vi "origin_distance (SubVI).vi"(8 "error in (no error)":errorcluster, 9 "Image Dst":T1, 10 "Origin Pixel":cluster{"X":sgl, "Y":sgl}, 11 "Image Src":T1) -> (0 "error out":errorcluster, 1 "Number of Particles":i32, 2 "Array":string[](array[string]), 3 "Array of Real World Coordinates":cluster{"X":sgl, "Y":sgl}[](array[cluster]), 5 "Image Out":T1)   [LabVIEW 2020]
uses:
  <vilib>/vision/Image Controls.llb/IMAQ Image.ctl
  <vilib>/vision/NI_Vision_Development_Module.lvlib
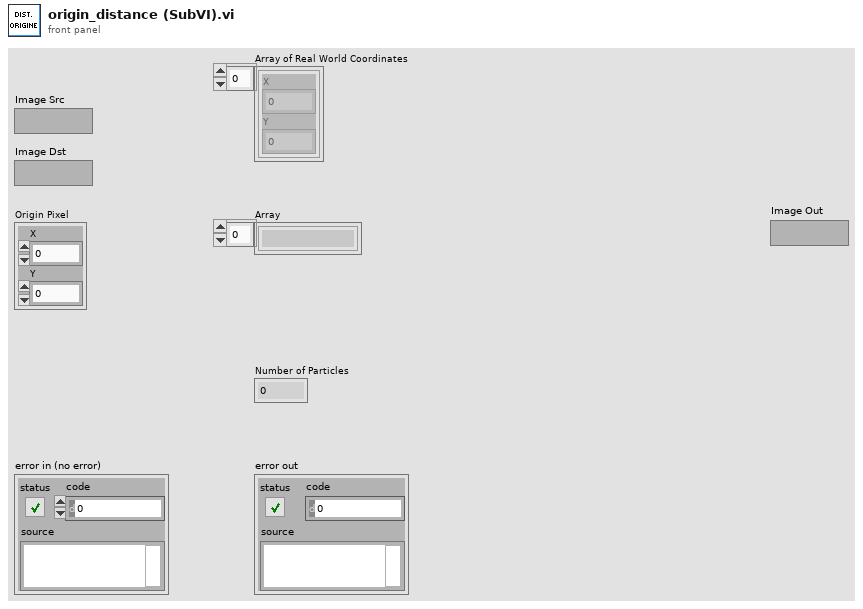
[diagram p1: front panel]
types:
  T1 = typedef "IMAQ Image.ctl" = refnum<image>
  T2 = cluster{"Area":dbl, "Number of Holes":dbl, "Bounding Rect":cluster{"Left":dbl, "Top":dbl, "Right":dbl, "Bottom":dbl}, "Center of Mass":cluster{"X":dbl, "Y":dbl}, "Orientation":dbl, "Dimensions":cluster{"Width":dbl, "Height":dbl}}[]
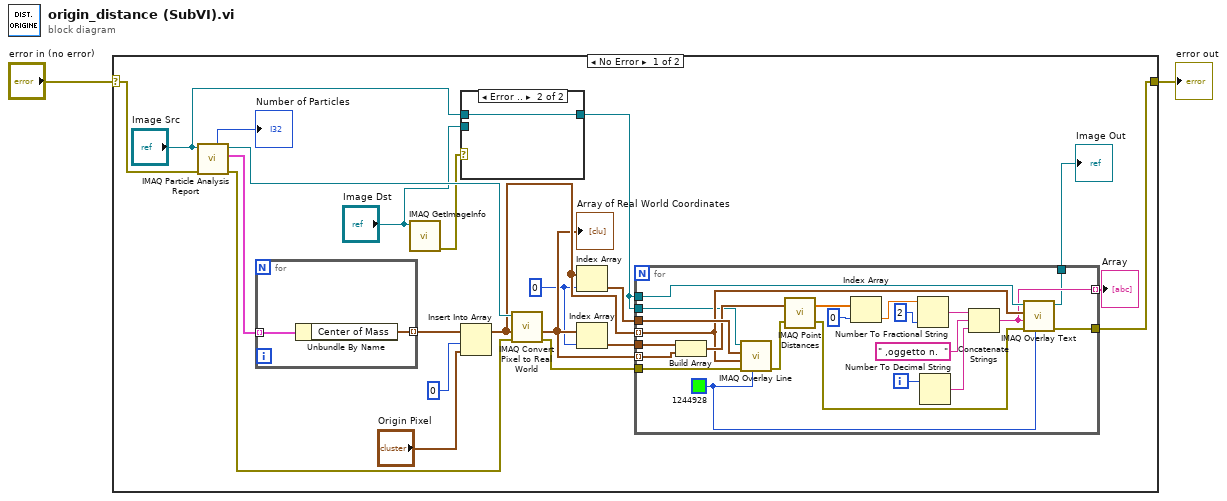
[diagram p0: block diagram]
diagram:
  n1 = case shown="No Error" "error in (no error)" {
    selector: "error in (no error)" -> [w9 w50]
    tunnel: [w8 w50] -> w1
    frame No Error {
      w12 = 0 ("index")
      n2 = call "IMAQ Particle Analysis Report"("error in (no error)"=w9, "Image"="Image Src") -> ("error out"=w21:errorcluster, "Particle Reports (Pixels)"=w19:T2, "Image Out (duplicate)"=w20:T1, "Number of Particles"=→"Number of Particles":i32)  [unwired: 4 in, 2 out]
      n3 = for {
        tunnel: [w48] -> w15 mode=indexing
        tunnel: w19 -> [w49] mode=indexing
        n4 = Unbundle By Name(w49) -> ("Center of Mass"=w48:cluster{"X":dbl, "Y":dbl})
      }
      n5 = call "IMAQ GetImageInfo"("Image"="Image Dst") -> ("error out"=w7:errorcluster)  [unwired: 3 in, 7 out]
      n6 = case shown="Error .." w7 {
        tunnel: "Image Dst" -> [w24 _]
        tunnel: [w24 w25] -> w5
        tunnel: "Image Src" -> [_ w25]
        frame No Error {
        }
        frame Error {
        }
      }
      n7 = Insert Into Array(array=w15, index=0, new element="Origin Pixel") -> (w16:cluster{"X":dbl, "Y":dbl}[])
      n8 = call "IMAQ Convert Pixel to Real World"("error in (no error)"=w21, "Array of Pixel Coordinates"=w16, "Calibrated Image"=w20) -> ("error out"=w22:errorcluster, "Array of Real World Coordinates"=w14:cluster{"X":sgl, "Y":sgl}[])  [unwired: 3 in, 4 out]
      "Array of Real World Coordinates" <- w14
      n9 = Index Array(array=w16, index=w12) -> (element=w11:cluster{"X":dbl, "Y":dbl})
      n10 = Index Array(array=w14, index=w12) -> (element=w13:cluster{"X":sgl, "Y":sgl})
      n11 = for {
        tunnel: w16 -> [w41] mode=indexing
        tunnel: w11 -> [w47]
        tunnel: w13 -> [w44]
        tunnel: w14 -> [w42] mode=indexing
        tunnel: [w45] -> w8
        tunnel: w5 -> [w30]
        tunnel: w5 -> [w29]
        tunnel: w22 -> [w28]
        tunnel: [w27] -> w23 mode=indexing
        tunnel: [w26] -> w3
        i -> [w36]
        w40 = u32 1244928 ("Color")
        n12 = Build Array(w44, w42) -> (w43:cluster{"X":sgl, "Y":sgl}[])
        n13 = call "IMAQ Overlay Line"("Color"=w40, "error in (no error)"=w28, "End Point"=w41, "Start Point"=w47, "Image"=w29) -> ("error out"=w46:errorcluster)  [unwired: 5 in, 1 out]
        n14 = call "IMAQ Point Distances"("Points"=w43, "error in (no error)"=w46) -> ("Distances"=w39:sgl[], "error out"=w32:errorcluster)  [unwired: 3 in]
        n15 = Index Array(array=w39, index=0) -> (element=w37:sgl)
        n16 = Number To Fractional String(number=w37, precision (6)=i16 2) -> (F-format string=w34:string)  [unwired: 2 in]
        n17 = Number To Decimal String(number=w36) -> (decimal integer string=w35:string)  [unwired: 1 in]
        n18 = Concatenate Strings(w34, " ,oggetto n.  " ("string"), w35) -> (w27:string)
        n19 = call "IMAQ Overlay Text"("Text Color (black)"=w40, "error in (no error)"=w32, "String"=w27, "Origin"=w41, "Image"=w30) -> ("error out"=w45:errorcluster, "Image Out"=w26:T1)  [unwired: 5 in]
      }
      "Array" <- w23
      "Image Out" <- w3
    }
    frame Error {
    }
  }
  "error out" <- w1
